vi "BasicExampleExportCSV.vi"() -> ()   [LabVIEW 2025]
uses:
  PalmSens/PalmSens.lvclass
  E:/PSCode/PalmSens_SDK/labview/PalmSens/Libraries/PalmSens.Core.Simplified.LabVIEW.dll
  PalmSens/Libraries/PalmSens.Core.Simplified.LabVIEW.dll
  <vilib>/Utility/file.llb/Write Delimited Spreadsheet (DBL).vi
panel:
  out "LSV Method Indicator":refnum<k24>
  out "Array":string[](array[string])
  out "Is Measuring":bool
  in  "PalmSens.lvclass":refnum<class "PalmSens.lvclass">
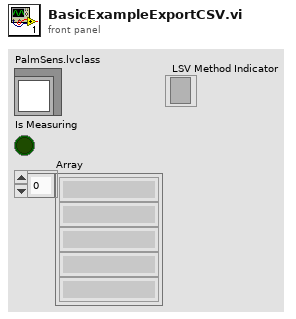
[diagram p1: front panel]
types:
  T1 = enum16{"open", "replace", "create", "open or create", "replace or create", "replace or create with confirmation"}
  T2 = typedef "MeasurementResults.ctl" = T3[]
  T3 = typedef "LiveCurveResult.ctl" = cluster{"X Label":string, "Y Label":string, "Name":string, "Index":i16, "Curve Values":cluster{"Values":cluster{"X Value":dbl, "Y Value":dbl}[], "Index":i16}}
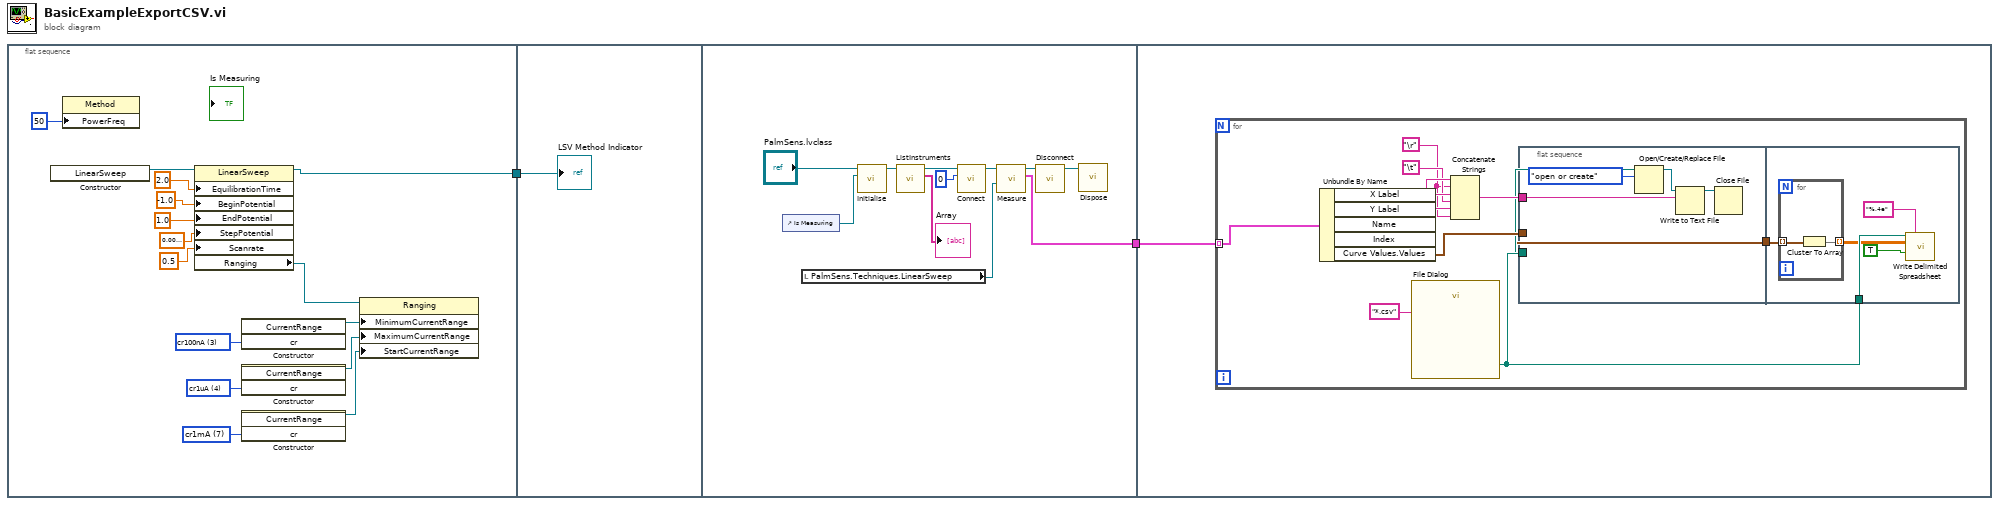
[diagram p0: block diagram]
diagram:
  n1 = flat-sequence {
    tunnel: [w3] -> w1
    tunnel: w1 -> [w18]
    tunnel: [w20] -> w2
    tunnel: w2 -> [w30]
    frame #0 {
      w6 = 4 items=["cr100pA"=0, "cr1nA"=1, "cr10nA"=2, "cr100nA"=3, "cr1uA"=4, "cr10uA"=5, "cr100uA"=6, "cr1mA"=7, "cr10mA"=8, "cr100mA"=9, "cr2uA"=10, "cr4uA"=11, "cr8uA"=12, "cr16uA"=13, "cr32uA"=14, "cr125uA"=17, "cr250uA"=18, "cr500uA"=19, "cr5mA"=20, "cr6uA"=21, "cr13uA"=22, "cr25uA"=23, "cr50uA"=24, "cr200uA"=25, "cr63uA"=26] ("cr")
      w5 = 7 items=["cr100pA"=0, "cr1nA"=1, "cr10nA"=2, "cr100nA"=3, "cr1uA"=4, "cr10uA"=5, "cr100uA"=6, "cr1mA"=7, "cr10mA"=8, "cr100mA"=9, "cr2uA"=10, "cr4uA"=11, "cr8uA"=12, "cr16uA"=13, "cr32uA"=14, "cr125uA"=17, "cr250uA"=18, "cr500uA"=19, "cr5mA"=20, "cr6uA"=21, "cr13uA"=22, "cr25uA"=23, "cr50uA"=24, "cr200uA"=25, "cr63uA"=26] ("cr")
      w4 = 3 items=["cr100pA"=0, "cr1nA"=1, "cr10nA"=2, "cr100nA"=3, "cr1uA"=4, "cr10uA"=5, "cr100uA"=6, "cr1mA"=7, "cr10mA"=8, "cr100mA"=9, "cr2uA"=10, "cr4uA"=11, "cr8uA"=12, "cr16uA"=13, "cr32uA"=14, "cr125uA"=17, "cr250uA"=18, "cr500uA"=19, "cr5mA"=20, "cr6uA"=21, "cr13uA"=22, "cr25uA"=23, "cr50uA"=24, "cr200uA"=25, "cr63uA"=26] ("cr")
      n2 = constructor class="LinearSweep"() -> (reference out=w14:refnum<k24>)  [unwired: 3 in, 2 out]
      n3 = property class="Method"("PowerFreq"=50) -> ()  [unwired: 2 in, 2 out]
      n4 = property class="LinearSweep"(reference=w14, "EquilibrationTime"=sgl 2.0, "BeginPotential"=sgl -1.0, "EndPotential"=sgl 1.0, "StepPotential"=sgl 0.01, "Scanrate"=sgl 0.5) -> (reference out=w3:refnum<k24>, "Ranging"=w17:refnum<k24>)  [unwired: 1 in, 1 out]
      n5 = constructor class="CurrentRange"("cr"=w4) -> (reference out=w13:refnum<k24>)  [unwired: 3 in, 3 out]
      n6 = constructor class="CurrentRange"("cr"=w6) -> (reference out=w15:refnum<k24>)  [unwired: 3 in, 3 out]
      n7 = constructor class="CurrentRange"("cr"=w5) -> (reference out=w16:refnum<k24>)  [unwired: 3 in, 3 out]
      n8 = property class="Ranging"(reference=w17, "MinimumCurrentRange"=w13, "MaximumCurrentRange"=w15, "StartCurrentRange"=w16) -> ()  [unwired: 1 in, 2 out]
    }
    frame #1 {
      "LSV Method Indicator" <- w18
    }
    frame #2 {
      n9 = control-ref of="Is Measuring"() -> (w26:refnum<vi>)
      n10 = local read "LSV Method Indicator"() -> (w23:refnum<k24>)
      n11 = call-dynamic "Initialise.vi"("Is Measuring Refnum"=w26, "PalmSens in"="PalmSens.lvclass") -> ("PalmSens out"=w27:refnum<class "PalmSens.lvclass">)  [unwired: 8 in, 1 out]
      n12 = call-dynamic "ListInstruments.vi"("PalmSens in"=w27) -> ("Array"=→"Array":string[], "PalmSens out"=w29:refnum<class "PalmSens.lvclass">)  [unwired: 8 in, 1 out]
      n13 = call-dynamic "Connect.vi"("Instrument Index"=0, "PalmSens in"=w29) -> ("PalmSens out"=w22:refnum<class "PalmSens.lvclass">)  [unwired: 8 in, 1 out]
      n14 = call-dynamic "Measure.vi"("Method .NET Refnum"=w23, "PalmSens in"=w22) -> ("Curves"=w20:T2, "PalmSens out"=w21:refnum<class "PalmSens.lvclass">)  [unwired: 2 in, 2 out]
      n15 = call-dynamic "Disconnect.vi"("PalmSens in"=w21) -> ("PalmSens out"=w19:refnum<class "PalmSens.lvclass">)  [unwired: 9 in, 1 out]
      n16 = call-dynamic "Dispose.vi"("PalmSens in"=w19) -> ()  [unwired: 9 in, 2 out]
    }
    frame #3 {
      n17 = for {
        tunnel: w30 -> [w32] mode=indexing
        w33 = "\r"
        n18 = Unbundle By Name(w32) -> ("X Label"=w40:string, "Y Label"=w38:string, "Name"=w41:string, "Curve Values.Values"=w31:cluster{"X Value":dbl, "Y Value":dbl}[])  [unwired: 1 out]
        n19 = call "File Dialog"("pattern (all files)"="*.csv") -> ("selected path"=w35:path)  [unwired: 11 in, 3 out]
        n20 = Concatenate Strings(w41, w33, w40, "\t", w38, w33) -> (w36:string)
        n21 = flat-sequence {
          tunnel: [w42] -> w37
          tunnel: w36 -> [w45]
          tunnel: w35 -> [w43]
          tunnel: w31 -> [w42]
          tunnel: w35 -> [w52]
          tunnel: w37 -> [w51]
          frame #0 {
            n22 = Open/Create/Replace File(file path (use dialog)=w43, operation (0:open)=T1."open or create") -> (refnum out=w46:refnum<file>)  [unwired: 4 in, 2 out]
            n23 = Write to Text File(file (use dialog)=w46, text=w45) -> (refnum out=w47:refnum<file>)  [unwired: 2 in, 2 out]
            n24 = Close File(refnum=w47) -> ()  [unwired: 1 in, 2 out]
          }
          frame #1 {
            n25 = for {
              tunnel: w51 -> [w54] mode=indexing
              tunnel: [w53] -> w50 mode=indexing
              n26 = Cluster To Array(cluster=w54) -> (array=w53:dbl[])
            }
            n27 = call-poly <vilib>:"Write Delimited Spreadsheet.vi"("file path (dialog if empty)"=w52, "format (%.3f)"="%.4e", "2D data"=w50, "append to file? (new file:F)"=TRUE) -> ()  [unwired: 10 in, 2 out]
          }
        }
      }
    }
  }
